vi "Piston Directionality.vi"() -> ()   [LabVIEW 2022 SP3]
uses:
  <vilib>/Analysis/NI_AALBase.lvlib
panel:
  out "lambda (mm)":dbl
  out "Polar Plot":picture
  out "polar":cluster{dbl[], dbl[]}(graph)
  out "radians":cluster{dbl[], dbl[]}(graph)
  in  "freq (MHz)":dbl=20.0
  in  "width (mm)":dbl=0.2
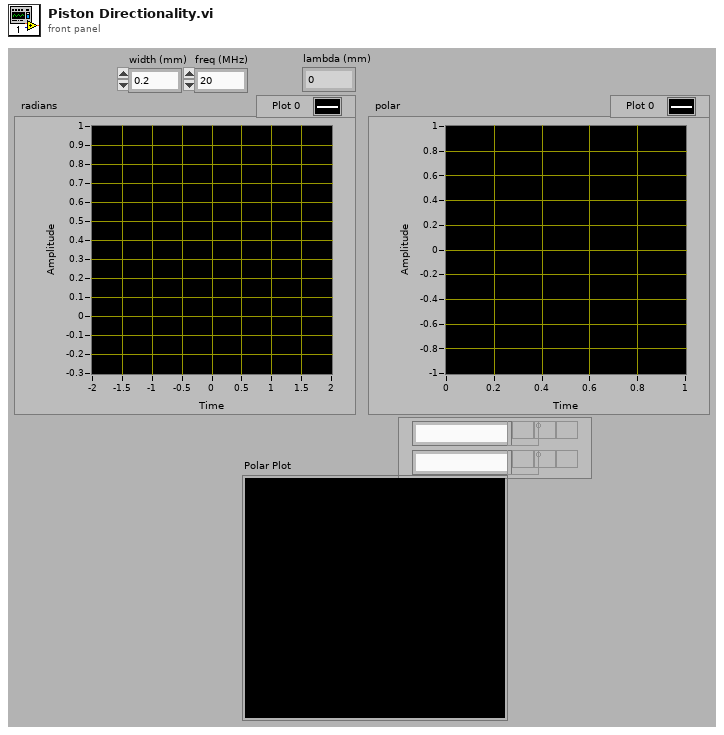
[diagram p1: front panel]
types:
  T1 = cluster{"maximum":dbl, "minimum":dbl, "clip to min":bool, "log?(F)":bool, "grid color":u32, "plot color":u32, "fmt and prec":cluster{"format":enum8{"Decimal", "Scientific", "Engineering", "Binary", "Octal", "Hex"}, "precision":u8}, "visible section":u16}
  T2 = typedef "LVBoundsTypeDef.ctl" = cluster{"Width":u32, "Height":u32}
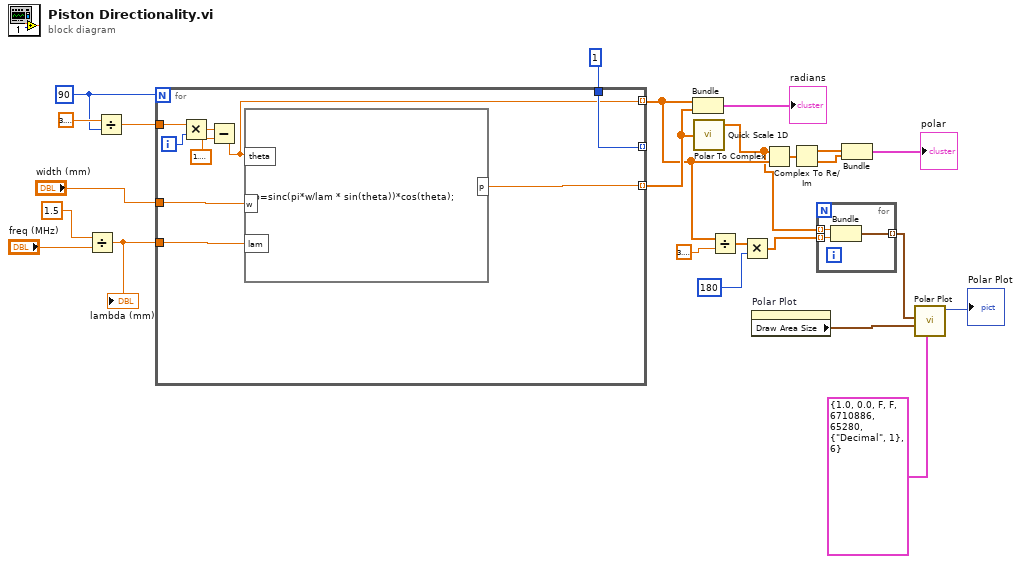
[diagram p0: block diagram]
diagram:
  w18 = 90
  n1 = Divide(x=1.5, y="freq (MHz)") -> (x/y=w22:dbl)
  "lambda (mm)" <- w22
  n2 = Divide(x=3.141592653589793, y=w18) -> (x/y=w17:dbl)
  n3 = for {
    N: w18 -> [_]
    tunnel: "width (mm)" -> [w33]
    tunnel: w22 -> [w32]
    tunnel: [w31] -> _ mode=indexing
    tunnel: 1 -> [w31]
    tunnel: w17 -> [w30]
    tunnel: [w26] -> w11 mode=indexing
    tunnel: [w25] -> w8 mode=indexing
    i -> [w29]
    n4 = Multiply(x=w30, y=w29) -> (x*y=w28:dbl)
    n5 = Subtract(x=w28, y=1.5707963267948966) -> (x-y=w25:dbl)
    n6 = formula code="p=sinc(pi*w/lam * sin(theta))*cos(theta);"("theta"=w25, "w"=w33, "lam"=w32) -> ("p"=w26:dbl)
  }
  n7 = Bundle(w8, w11) -> (→"radians":cluster{dbl[], dbl[]})  [unwired: 1 out]
  n8 = call <vilib>:"Quick Scale 1D.vi"("X"=w11) -> ("Y[i]=X[i]/Max|X|"=w4:dbl[])  [unwired: 2 out]
  n9 = Divide(x=w8, y=3.141592653589793) -> (x/y=w6:dbl[])
  n10 = Multiply(x=w6, y=180) -> (x*y=w3:dbl[])
  n11 = property on="Polar Plot" class="Pict"() -> ("Draw Area Size"=w10:T2)  [unwired: 2 in, 2 out]
  n12 = Polar To Complex(1:w8, 2:w4) -> (0:w15:cdb[])
  n13 = Complex To Re/Im(x + iy=w15) -> (x=w14:dbl[], y=w13:dbl[])
  n14 = for {
    tunnel: w4 -> [w36] mode=indexing
    tunnel: w3 -> [w35] mode=indexing
    tunnel: [w34] -> w2 mode=indexing
    n15 = Bundle(w36, w35) -> (w34:cluster{dbl, dbl})  [unwired: 1 out]
  }
  n16 = Bundle(w14, w13) -> (→"polar":cluster{dbl[], dbl[]})  [unwired: 1 out]
  n17 = call <vilib>:"Polar Plot.vi"("polar attributes"=T1 {"maximum"=1.0, "minimum"=0.0, "clip to min"=FALSE, "log?(F)"=FALSE, "grid color"=6710886, "plot color"=65280, "fmt and prec"={"format"=enum."Decimal", "precision"=1}, "visible section"=6}, "dimensions (w,h)"=w10, "data array [mag, phase (deg)]"=w2) -> ("new picture"=→"Polar Plot":picture)  [unwired: 1 in, 7 out]
